vi "CtrCntrl.vi"(10 "error in (no error)":errorcluster, 11 ".NET Refnum":refnum<k24>) -> (0 "InvertGate":bool, 1 "Recycle":bool, 2 "error out":errorcluster, 3 ".NET Refnum 2":refnum<k24>, 4 "OutputVal1":u64, 5 "MinLimit":u64, 6 "OutputVal0":u64, 7 "MaxLimit":u64, 8 "OutputOn":bool, 9 "RangeLimitOn":bool)   [LabVIEW 2010]
uses:
  C:/Program Files/National Instruments/LabVIEW 2010/vi.lib/ULx/ULx_LV.dll
  Program Files/National Instruments/LabVIEW 2010/vi.lib/ULx/ULx_LV.dll
panel:
  out "ClearOnRead":bool
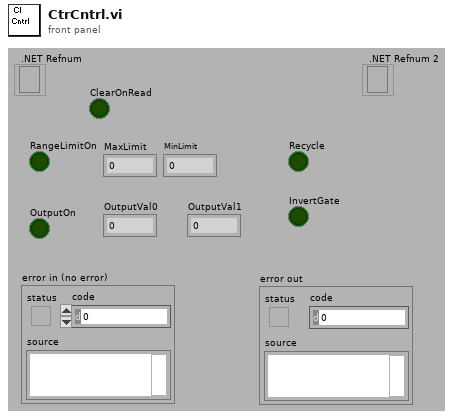
[diagram p1: front panel]
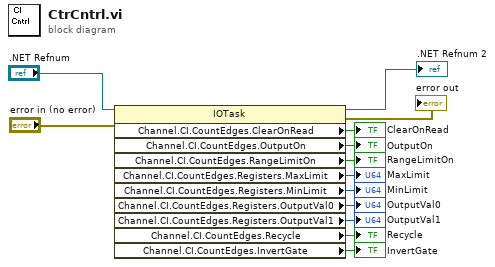
[diagram p0: block diagram]
diagram:
  n1 = property class="IOTask"(reference=".NET Refnum", error in="error in (no error)") -> (reference out=→".NET Refnum 2":refnum<k24>, error out=→"error out":errorcluster, "Channel.CI.CountEdges.ClearOnRead"=→"ClearOnRead":bool, "Channel.CI.CountEdges.OutputOn"=→"OutputOn":bool, "Channel.CI.CountEdges.RangeLimitOn"=→"RangeLimitOn":bool, "Channel.CI.CountEdges.Registers.MaxLimit"=→"MaxLimit":u64, "Channel.CI.CountEdges.Registers.MinLimit"=→"MinLimit":u64, "Channel.CI.CountEdges.Registers.OutputVal0"=→"OutputVal0":u64, "Channel.CI.CountEdges.Registers.OutputVal1"=→"OutputVal1":u64, "Channel.CI.CountEdges.Recycle"=→"Recycle":bool, "Channel.CI.CountEdges.InvertGate"=→"InvertGate":bool)
